vi "Example Launched Application.vi"(11 "Splash Notifier":refnum<notifier>) -> (0 "error out":errorcluster)   [LabVIEW 2020]
uses:
  TypeDefs/Init States_ENUM.ctl
  16738011-b86e-4325-95c2-9adcdd8569c0.vi
  <vilib>/LAVA/UI Tools/Fading/_Fade Out(I32)__lava_lib_ui_tools.vi
  <vilib>/LAVA/UI Tools/Fading/_Fade In(I32)__lava_lib_ui_tools.vi
  <vilib>/LAVA/UI Tools/Fading/SetTransparency(U8)__lava_lib_ui_tools.vi
panel:
  in  "Stop":bool
  out "Data":cluster{dbl, dbl}(graph)
  in  "Init State":T1
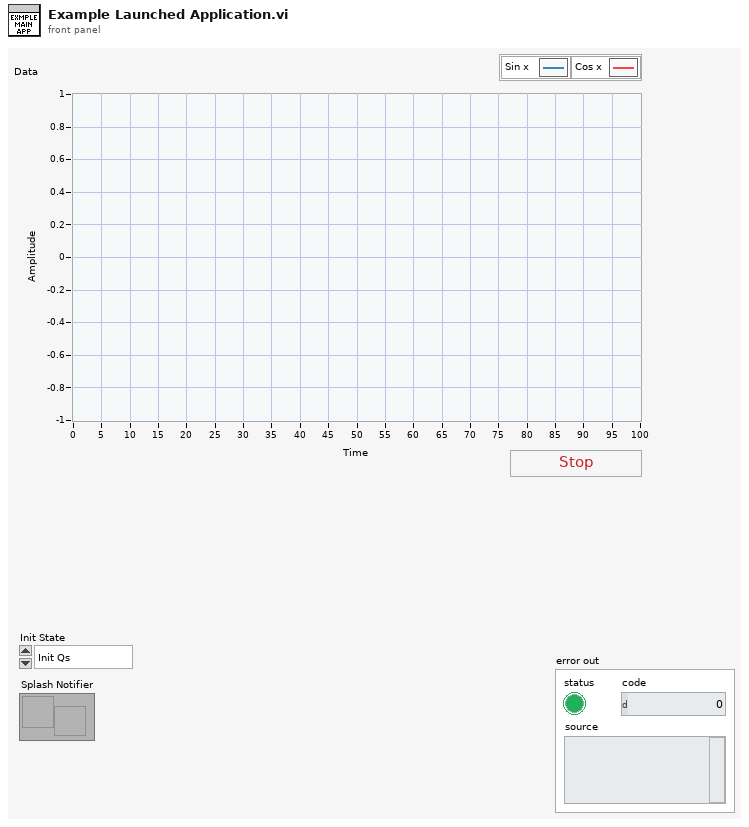
[diagram p1: front panel]
types:
  T1 = typedef "Init States_ENUM.ctl" = enum16{"Init Qs", "Init Logging", "Init User Events", "Init Instruments", "Init Comms", "Init Complete"}
  T2 = enum32{"Invalid", "Standard", "Closed", "Hidden", "Minimized", "Maximized"}
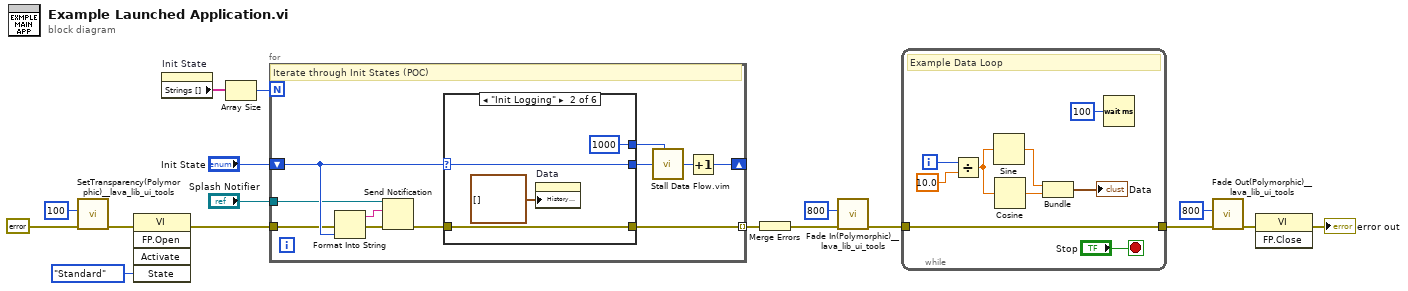
[diagram p0: block diagram]
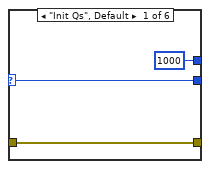
[diagram p2: hidden frame]
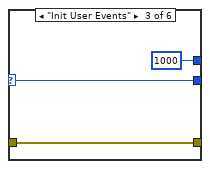
[diagram p3: hidden frame]
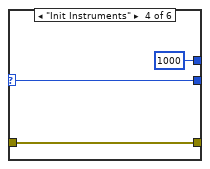
[diagram p4: hidden frame]
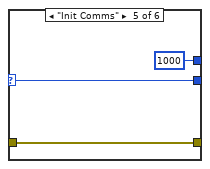
[diagram p5: hidden frame]
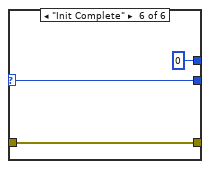
[diagram p6: hidden frame]
diagram:
  n1 = call-poly <vilib>:"SetTransparency(Polymorphic)__lava_lib_ui_tools.vi"("error in"=errorcluster {"status"=FALSE, "code"=0, "source"=""}, "Transparency (%)"=u8 100) -> ("error out"=w7:errorcluster)  [unwired: 8 in, 1 out]
  n2 = invoke class="VI" method="FP.Open"(error in=w7, "State"=T2."Standard") -> (error out=w3:errorcluster)  [unwired: 3 in, 4 out]
  n3 = property on="Init State" class="Enum (strict)"() -> ("Strings []"=w16:string[])  [unwired: 2 in, 2 out]
  n4 = Array Size(array=w16) -> (size(s)=w17:i32)
  n5 = for {
    N: w17 -> [_]
    shift-right: [w28] -> _
    shift-left: "Init State" -> [w27]
    tunnel: w3 -> [w26]
    tunnel: [w24] -> w15 mode=indexing
    tunnel: "Splash Notifier" -> [w23]
    # "Iterate through Init States (POC)"
    n6 = Format Into String(error in=w26, w27) -> (resulting string=w20:string, error out=w19:errorcluster)  [unwired: 2 in]
    n7 = Send Notification(notification=w20, notifier=w23, error in (no error)=w19) -> (error out=w25:errorcluster)  [unwired: 1 out]
    n8 = case shown="\"Init Logging\"" w27 {
      selector: w27 -> [w30 w35 w38 w41 w44 w46]
      tunnel: [w30 w35 w38 w41 w44 w46] -> w22
      tunnel: w25 -> [w31 w34 w37 w40 w43 w47]
      tunnel: [w31 w34 w37 w40 w43 w47] -> w24
      tunnel: [u32 1000 ("milliseconds to wait") u32 1000 ("milliseconds to wait") u32 1000 ("milliseconds to wait") u32 1000 ("milliseconds to wait") u32 1000 ("milliseconds to wait") u32 0 ("milliseconds to wait")] -> w18
      frame "Init Qs", Default {
      }
      frame "Init Logging" {
        n9 = property on="Data" class="WFChart (strict)"("History Data"=cluster{dbl, dbl}[] []) -> ()  [unwired: 2 in, 2 out]
      }
      frame "Init User Events" {
      }
      frame "Init Instruments" {
      }
      frame "Init Comms" {
      }
      frame "Init Complete" {
      }
    }
    n10 = call "Stall Data Flow.vim"("value in"=w22, "milliseconds to wait"=w18) -> ("value out"=w21:T1)  [unwired: 1 out]
    n11 = Increment(x=w21) -> (x+1=w28:T1)
  }
  n12 = Merge Errors(w15) -> (w12:errorcluster)
  n13 = call-poly <vilib>:"Fade In(Polymorphic)__lava_lib_ui_tools.vi"("error in"=w12, "Fade time (ms)"=800) -> ("error out"=w11:errorcluster)  [unwired: 8 in, 1 out]
  n14 = while {
    tunnel: w11 -> [w48]
    tunnel: [w48] -> w9
    i -> [w50]
    stop <- "Stop" stop-if-true
    # "Example Data Loop"
    n15 = Divide(x=w50, y=10.0) -> (x/y=w54:dbl)
    n16 = Sine(x=w54) -> (sin(x)=w52:dbl)
    n17 = Cosine(x=w54) -> (cos(x)=w53:dbl)
    n18 = Bundle(w52, w53) -> (→"Data":cluster{dbl, dbl})  [unwired: 1 in]
    n19 = Wait (ms)(milliseconds to wait=u32 100) -> ()  [unwired: 1 out]
  }
  n20 = call-poly <vilib>:"Fade Out(Polymorphic)__lava_lib_ui_tools.vi"("error in"=w9, "Fade time (ms)"=800) -> ("error out"=w2:errorcluster)  [unwired: 8 in, 1 out]
  n21 = invoke class="VI" method="FP.Close"(error in=w2) -> (error out=→"error out":errorcluster)  [unwired: 2 in, 2 out]
